vi "Convert to Part 2.vi"(11 "Puzzle 15-1":T1) -> (3 "Puzzle 15-2":T1)   [LabVIEW 2020]
uses:
  Part 1/Puzzle 15-1.ctl
  Part 1/Position.ctl
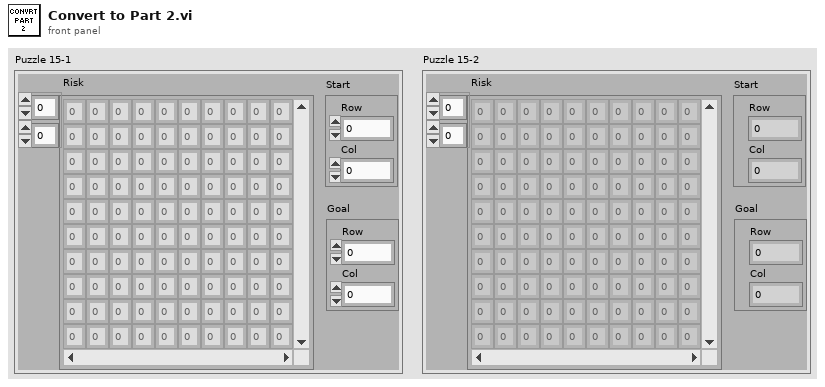
[diagram p1: front panel]
types:
  T1 = typedef "Puzzle 15-1.ctl" = cluster{"Risk":i32[][], "Start":T2, "Goal":T2}
  T2 = typedef "Position.ctl" = cluster{"Row":i32, "Col":i32}
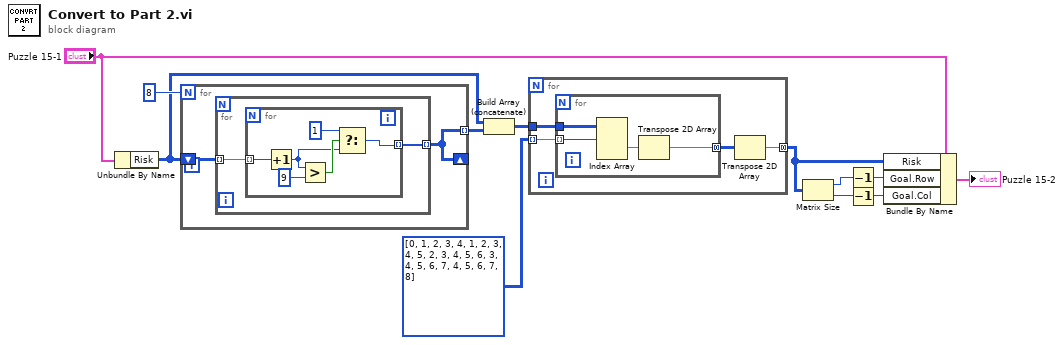
[diagram p0: block diagram]
diagram:
  n1 = Unbundle By Name("Puzzle 15-1") -> ("Risk"=w8:i32[][])
  n2 = for {
    N: 8 -> [_]
    tunnel: [w13] -> w10 mode=indexing
    shift-right: [w13] -> _
    shift-left: w8 -> [w14]
    n3 = for {
      tunnel: w14 -> [w16] mode=indexing
      tunnel: [w15] -> w13 mode=indexing
      n4 = for {
        tunnel: w16 -> [w22] mode=indexing
        tunnel: [w17] -> w15 mode=indexing
        n5 = Increment(x=w22) -> (x+1=w19:i32)
        n6 = Greater?(x=w19, y=9) -> (0:w20:bool)
        n7 = Select(t=1, s=w20, f=w19) -> (s? t:f=w17:i32)
      }
    }
  }
  n8 = Build Array (concatenate)(w8, w10) -> (w9:i32[][][])
  n9 = for {
    tunnel: w9 -> [w26]
    tunnel: i32[][] [[0, 1, 2, 3, 4], [1, 2, 3, 4, 5], [2, 3, 4, 5, 6], [3, 4, 5, 6, 7], [4, 5, 6, 7, 8]] -> [w25] mode=indexing
    tunnel: [w23] -> w5 mode=concatenating
    n10 = for {
      tunnel: w26 -> [w30]
      tunnel: w25 -> [w29] mode=indexing
      tunnel: [w27] -> w24 mode=concatenating
      n11 = Index Array(array=w30, index (dim 0)=w29) -> (element=w28:i32[][])  [unwired: 2 in]
      n12 = Transpose 2D Array(2D array=w28) -> (transposed array=w27:i32[][])
    }
    n13 = Transpose 2D Array(2D array=w24) -> (transposed array=w23:i32[][])
  }
  n14 = Matrix Size(0:w5) -> (1:w3:i32, 2:w2:i32)
  n15 = Decrement(x=w3) -> (x-1=w4:i32)
  n16 = Decrement(x=w2) -> (x-1=w1:i32)
  n17 = Bundle By Name(cluster="Puzzle 15-1", "Risk"=w5, "Goal.Row"=w4, "Goal.Col"=w1) -> (→"Puzzle 15-2":T1)
